vi "Ducat_AutoSearch.vi"(8 "error in":errorcluster) -> (0 "error out":errorcluster, 3 "Ducat Number":string)   [LabVIEW 2011]
doc: "This VI automatically determines the ducat that's connected to the current tester platform by reading in the testers.txt file and pinging each ducat listed until a response is found.\n\nInputs:\nNone\n\nOutputs:\n1. Ducat Nubmer: Number of the ducat attached to the tester platform (ducat 3, etc.)"
uses:
  <vilib>/Utility/error.llb/DialogType.ctl
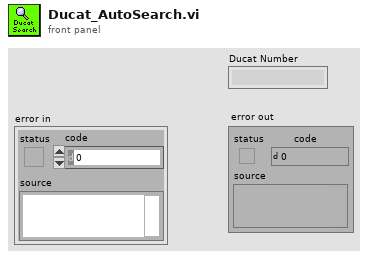
[diagram p1: front panel]
types:
  T1 = enum16{"open", "replace", "create", "open or create", "replace or create", "replace or create with confirmation"}
  T2 = typedef "DialogType.ctl" = u16
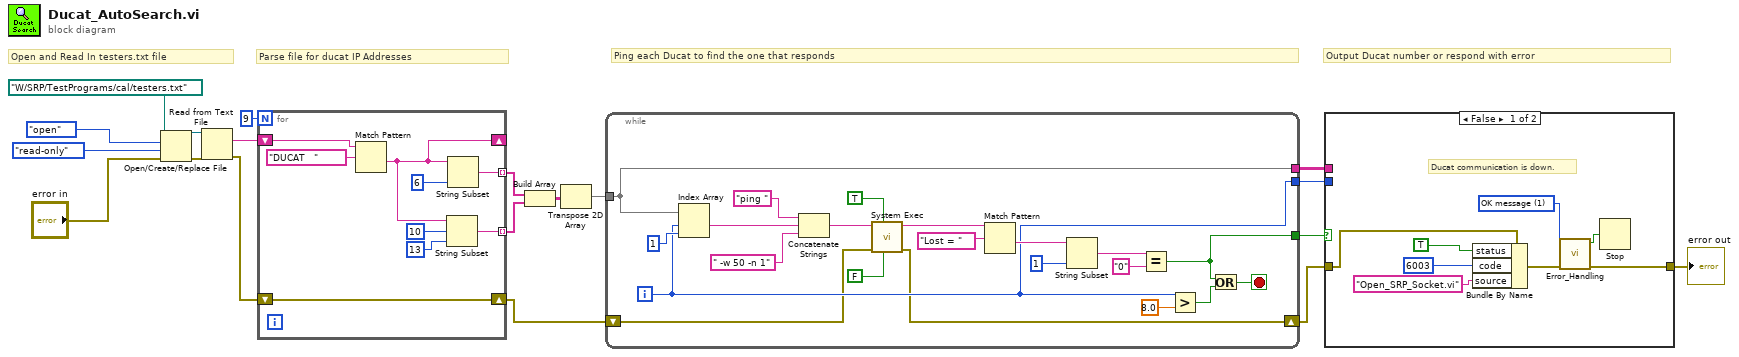
[diagram p0: block diagram]
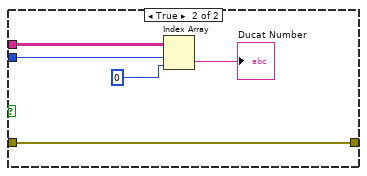
[diagram p2: hidden frame]
diagram:
  # "Output Ducat number or respond with error"
  # "Ping each Ducat to find the one that responds"
  # "Parse file for ducat IP Addresses"
  # "Open and Read In testers.txt file"
  n1 = Open/Create/Replace File(file path (use dialog)=path "W:/SRP/TestPrograms/cal/testers.txt", error in="error in", operation (0:open)=T1."open", access (0:read/write)=enum16{"read/write", "read-only", "write-only"}."read-only") -> (refnum out=w19:refnum<file>, error out=w9:errorcluster)  [unwired: 2 in, 1 out]
  n2 = Read from Text File(file (use dialog)=w19, error in=w9) -> (text=w14:string, error out=w7:errorcluster)  [unwired: 2 in, 2 out]
  n3 = for {
    N: 9 -> [_]
    tunnel: [w27] -> w13 mode=indexing
    shift-right: [w25] -> _
    shift-left: w14 -> [w26]
    tunnel: [w24] -> w12 mode=indexing
    shift-right: [w20] -> w6
    shift-left: w7 -> [w20]
    n4 = Match Pattern(string=w26, regular expression="DUCAT   ") -> (after substring=w25:string)  [unwired: 1 in, 3 out]
    n5 = String Subset(string=w25, offset (0)=10, length (rest)=13 ("length (rest)")) -> (substring=w24:string)
    n6 = String Subset(string=w25, length (rest)=6 ("length (rest)")) -> (substring=w27:string)  [unwired: 1 in]
  }
  n7 = Build Array(w13, w12) -> (w11:string[][])
  n8 = Transpose 2D Array(2D array=w11) -> (transposed array=w10:string[][])
  n9 = while {
    tunnel: w10 -> [w36]
    tunnel: [w36] -> w5
    tunnel: [w32] -> w4
    shift-right: [w30] -> w1
    shift-left: w6 -> [w31]
    tunnel: [w29] -> w3
    i -> [w32]
    stop <- w34 stop-if-true
    n10 = Index Array(array=w36, index (row)=w32, index (col)=1 ("disabled index (col)")) -> (element=w43:string)
    n11 = Concatenate Strings("ping " ("regular expression"), w43, " -w 50 -n 1" ("regular expression")) -> (w44:string)
    n12 = call <vilib>:"System Exec.vi"("run minimized? (F)"=FALSE, "wait until completion? (T)"=TRUE, "error in (no error)"=w31, "command line"=w44) -> ("error out"=w30:errorcluster, "standard output"=w41:string)  [unwired: 4 in, 2 out]
    n13 = Match Pattern(string=w41, regular expression="Lost = ") -> (after substring=w39:string)  [unwired: 1 in, 3 out]
    n14 = String Subset(string=w39, length (rest)=1 ("length (rest)")) -> (substring=w38:string)  [unwired: 1 in]
    n15 = Equal?(x=w38, y="0") -> (x = y?=w29:bool)
    n16 = Greater?(x=w32, y=8.0) -> (0:w35:bool)
    n17 = Or(x=w29, y=w35) -> (x .or. y?=w34:bool)
  }
  n18 = case shown="False" w3 {
    tunnel: w5 -> [_ w61]
    tunnel: w4 -> [_ w60]
    tunnel: [w53 w58] -> w2
    tunnel: w1 -> [w54 w58]
    frame False {
      w51 = T2 1 items=["no dialog", "OK message", "continue or stop message", "OK message + warnings", "continue/stop + warnings"] ("type of dialog (OK msg:1)")
      # "Ducat communication is down."
      n19 = Bundle By Name(cluster=w54, "status"=TRUE, "code"=6003, "source"="Open_SRP_Socket.vi") -> (w52:errorcluster)
      n20 = call "Error_Handling.vi"("error in (no error)"=w52, "type of dialog (OK msg:1)"=w51) -> ("error out"=w53:errorcluster, "error?"=w50:bool)  [unwired: 8 in]
      n21 = Stop(stop? (T)=w50) -> ()
    }
    frame True {
      n22 = Index Array(array=w61, index (row)=w60, index (col)=0 ("disabled index (col)")) -> (element=→"Ducat Number":string)
    }
  }
  "error out" <- w2
